vi "IO Read.vi"(11 "I/O":refnum<k21>) -> (3 "data":bool)   [LabVIEW 2017, in "HD44780 FPGA.lvlib"]
uses:
  HD44780 FPGA.lvlib
  <vilib>/rvi/eio/common/nirviEmuTemplateMethod_errors.vi
  <vilib>/eio/EIONode/EIONode.xnode
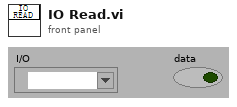
[diagram p1: front panel]
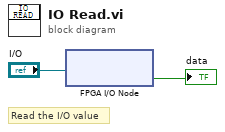
[diagram p0: block diagram]
diagram:
  # "Read the I/O value"
  n1 = xnode "FPGA I/O Node"("FPGA I/O In"="I/O") -> ("I/O Item"=→"data":bool)  [unwired: 1 out]
